vi "Combine Data.vi"() -> ()   [LabVIEW 2010]
panel:
  out "before substring":string
  out "after substring":string
  out "selected path":path
  out "Array":string[](array[string])
  out "error out":errorcluster
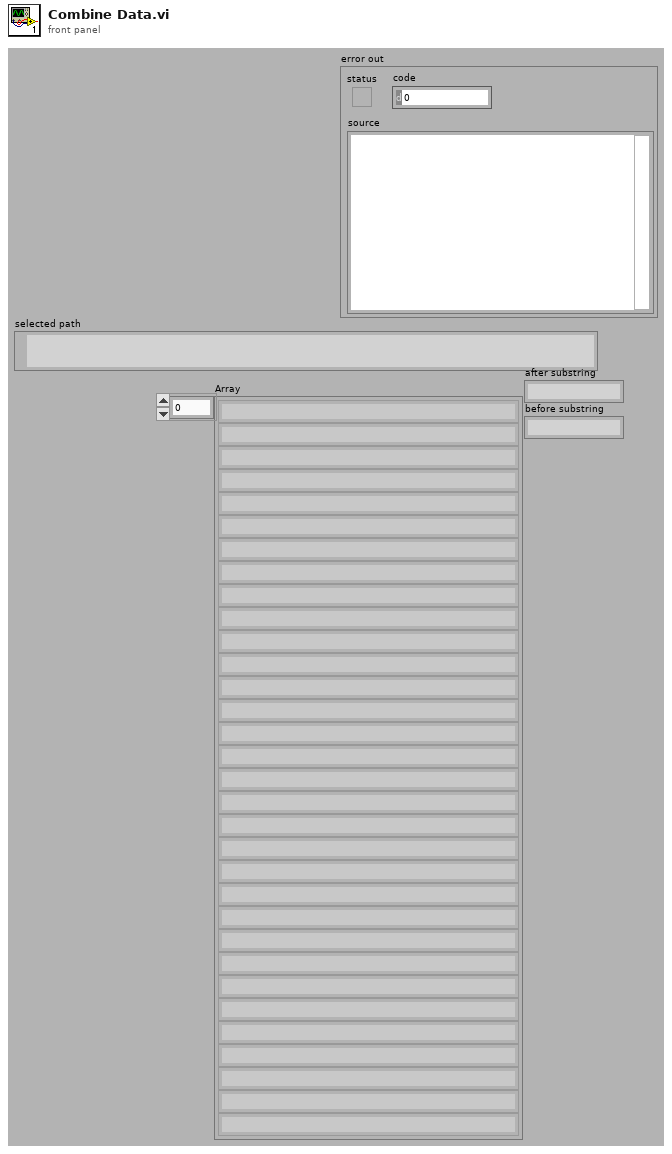
[diagram p1: front panel]
types:
  T1 = enum16{"open", "replace", "create", "open or create", "replace or create", "replace or create with confirmation"}
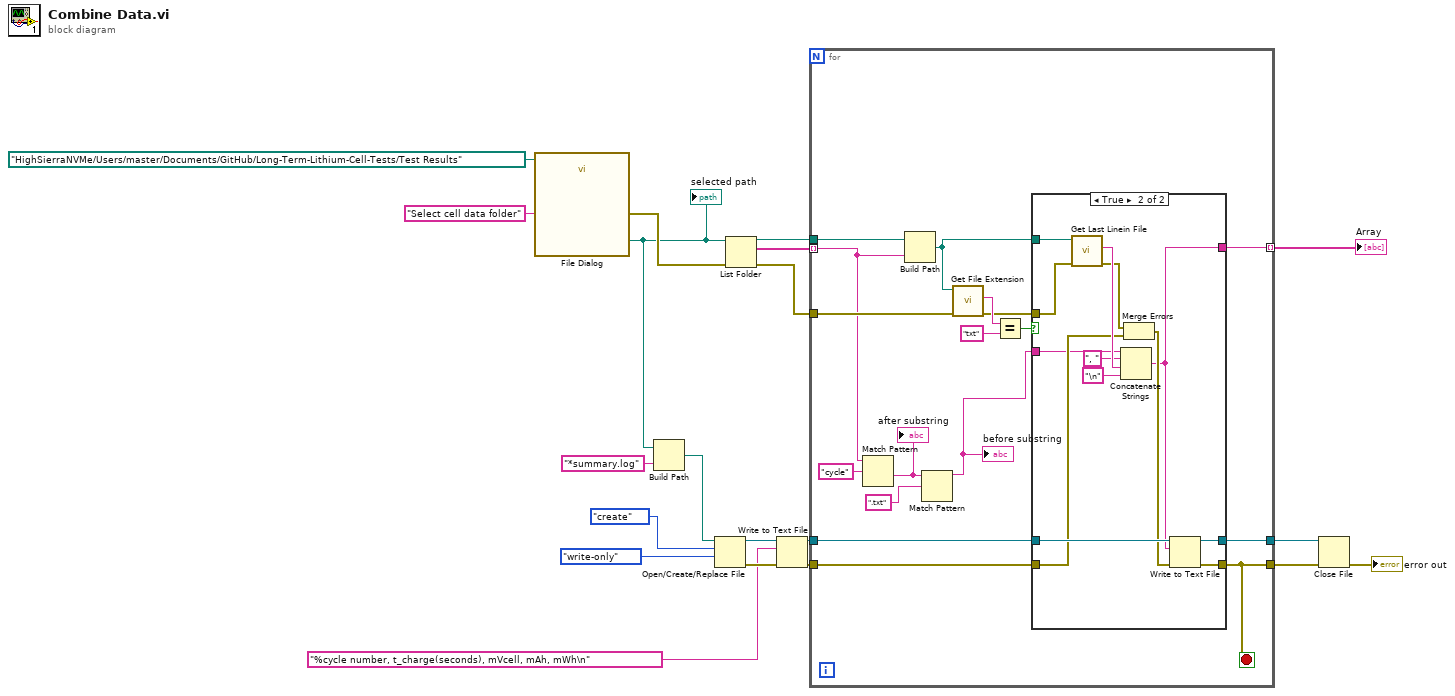
[diagram p0: block diagram]
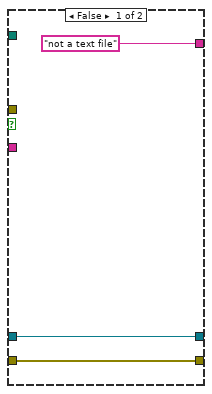
[diagram p2: hidden frame]
diagram:
  n1 = call "File Dialog"("start path"=path "/HighSierraNVMe/Users/master/Documents/GitHub/Long-Term-Lithium-Cell-Tests/Test Results", "prompt"="Select cell data folder") -> ("selected path"=w12:path, "error out"=w17:errorcluster)  [unwired: 10 in, 2 out]
  "selected path" <- w12
  n2 = Build Path(base path=w12, name or relative path="*summary.log") -> (appended path=w10:path)
  n3 = Open/Create/Replace File(file path (use dialog)=w10, operation (0:open)=T1."create", access (0:read/write)=enum16{"read/write", "read-only", "write-only"}."write-only") -> (refnum out=w5:refnum<file>, error out=w4:errorcluster)  [unwired: 3 in, 1 out]
  n4 = List Folder(path=w12, error in=w17) -> (path out=w19:path, filenames=w18:string[], error out=w16:errorcluster)  [unwired: 2 in, 1 out]
  n5 = Write to Text File(file (use dialog)=w5, text="%cycle number, t_charge(seconds), mVcell, mAh, mWh\n", error in=w4) -> (refnum out=w2:refnum<file>, error out=w3:errorcluster)  [unwired: 1 in, 1 out]
  n6 = for {
    tunnel: w19 -> [w33]
    tunnel: w18 -> [w25] mode=indexing
    tunnel: w16 -> [w37]
    tunnel: [w30] -> w15 mode=indexing
    tunnel: w2 -> [w29]
    tunnel: w3 -> [w28]
    tunnel: [w27] -> w8
    tunnel: [w26] -> w7
    stop <- w26 stop-if-true
    n7 = Match Pattern(string=w25, regular expression="cycle") -> (after substring=w23:string)  [unwired: 1 in, 3 out]
    "after substring" <- w23
    n8 = Build Path(base path=w33, name or relative path=w25) -> (appended path=w31:path)
    n9 = Match Pattern(string=w23, regular expression=".txt") -> (before substring=w21:string)  [unwired: 1 in, 3 out]
    "before substring" <- w21
    n10 = call <vilib>:"Get File Extension.vi"("error in (no error)"=w37, "file"=w31) -> ("error out"=w32:errorcluster, "lowercase file extension"=w35:string)  [unwired: 6 in, 2 out]
    n11 = Equal?(x=w35, y="txt" ("x")) -> (x = y?=w34:bool)
    n12 = case shown="True" w34 {
      tunnel: w31 -> [_ w53]
      tunnel: w32 -> [_ w52]
      tunnel: ["not a text file" ("Last Line in File") w41] -> w30
      tunnel: w29 -> [w39 w49]
      tunnel: w28 -> [w38 w45]
      tunnel: [w39 w48] -> w27
      tunnel: [w38 w47] -> w26
      tunnel: w21 -> [_ w43]
      frame False {
      }
      frame True {
        n13 = call "Get Last Linein File.vi"("error in"=w52, "file path (use dialog)"=w53) -> ("error out"=w46:errorcluster, "Last Line in File"=w50:string)  [unwired: 8 in]
        n14 = Concatenate Strings(w43, ", " ("string"), w50, "\n" ("string")) -> (w41:string)
        n15 = Merge Errors(w46, w45) -> (w44:errorcluster)
        n16 = Write to Text File(file (use dialog)=w49, text=w41, error in=w44) -> (refnum out=w48:refnum<file>, error out=w47:errorcluster)  [unwired: 1 in, 1 out]
      }
    }
  }
  "Array" <- w15
  n17 = Close File(refnum=w8, error in=w7) -> (error out=→"error out":errorcluster)  [unwired: 1 out]
